vi "Array Subset.vi"() -> ()   [LabVIEW 2013]
panel:
  out "subarray":dbl[](array[numeric])
  in  "length":i32
  in  "index":i32
  in  "Array":dbl[](array[numeric])
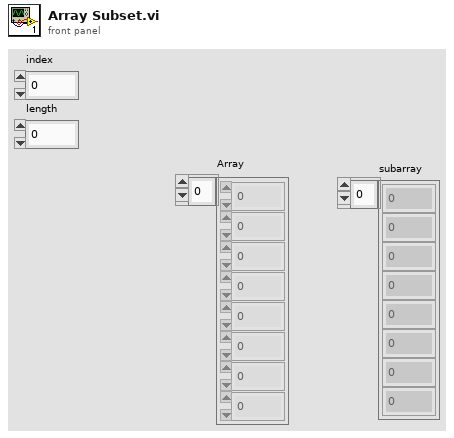
[diagram p1: front panel]
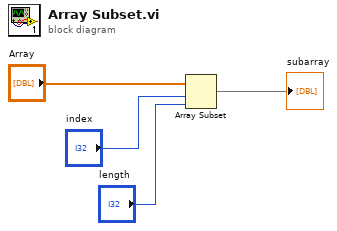
[diagram p0: block diagram]
diagram:
  n1 = Array Subset(array="Array", index="index", length="length") -> (→"subarray":dbl[])
